vi "MSE (SubVI).vi"(9 "Img":dbl[][](array[numeric]), 11 "Ref":dbl[][](array[numeric])) -> (3 "MSError":dbl)   [LabVIEW 2014]
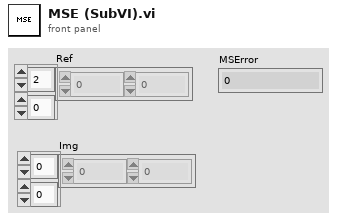
[diagram p1: front panel]
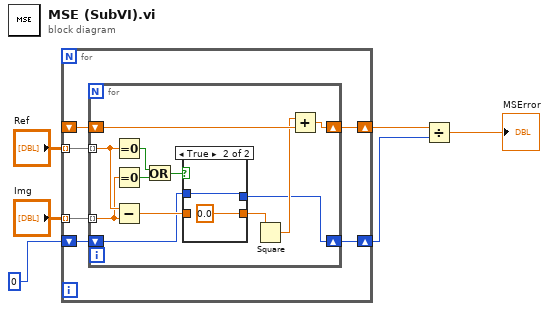
[diagram p0: block diagram]
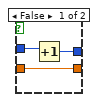
[diagram p2: hidden frame]
diagram:
  n1 = for {
    tunnel: "Ref" -> [w12] mode=indexing
    tunnel: "Img" -> [w11] mode=indexing
    shift-right: [w10] -> w3
    shift-left: _ -> [w9]
    shift-right: [w7] -> w1
    shift-left: 0 -> [w8]
    n2 = for {
      tunnel: w12 -> [w22] mode=indexing
      tunnel: w11 -> [w21] mode=indexing
      shift-right: [w23] -> w10
      shift-left: w9 -> [w24]
      shift-right: [w13] -> w7
      shift-left: w8 -> [w14]
      n3 = Equal To 0?(x=w22) -> (x = 0?=w19:bool)
      n4 = Equal To 0?(x=w21) -> (x = 0?=w20:bool)
      n5 = Subtract(x=w22, y=w21) -> (x-y=w17:dbl)
      n6 = Or(x=w19, y=w20) -> (x .or. y?=w18:bool)
      n7 = case shown="True" w18 {
        tunnel: w17 -> [w27 _]
        tunnel: [w27 0.0] -> w16
        tunnel: w14 -> [w26 w28]
        tunnel: [w25 w28] -> w13
        frame False {
          n8 = Increment(x=w26) -> (x+1=w25:i32)
        }
        frame True {
        }
      }
      n9 = Square(x=w16) -> (x^2=w15:dbl)
      n10 = Add(x=w15, y=w24) -> (x+y=w23:dbl)
    }
  }
  n11 = Divide(x=w3, y=w1) -> (x/y=→"MSError":dbl)
